vi "AbsMove.vi"(9 "Pos":dbl[](array[numeric]), 10 "error in":errorcluster) -> (2 "error out":errorcluster)   [LabVIEW 2022 SP3]
uses:
  Newport.XPS.CommandInterface
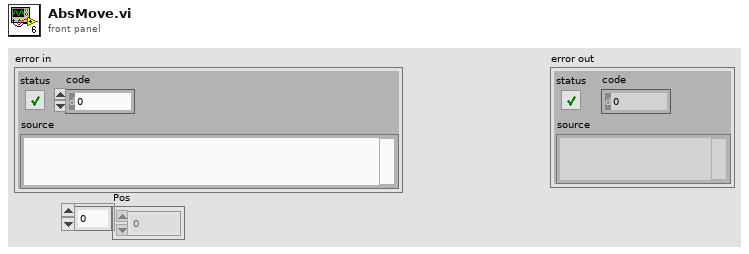
[diagram p1: front panel]
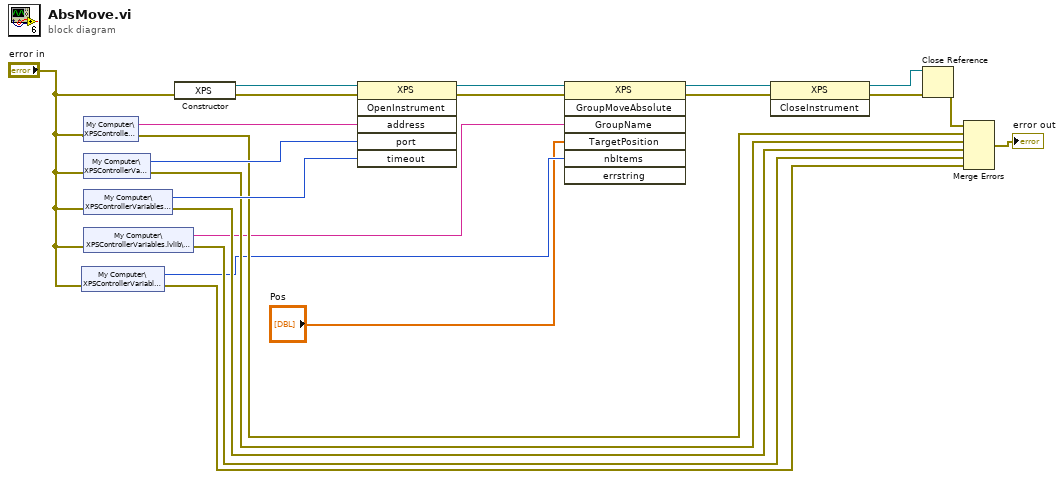
[diagram p0: block diagram]
diagram:
  n1 = shared-variable "My Computer\\XPSControllerVariables.lvlib\\nbitem"(error in="error in") -> (w4:i16, error out=w1:errorcluster)
  n2 = shared-variable "My Computer\\XPSControllerVariables.lvlib\\IP"(error in="error in") -> (w18:string, error out=w11:errorcluster)
  n3 = shared-variable "My Computer\\XPSControllerVariables.lvlib\\Port"(error in="error in") -> (w17:i16, error out=w10:errorcluster)
  n4 = shared-variable "My Computer\\XPSControllerVariables.lvlib\\Timeout"(error in="error in") -> (w16:i16, error out=w9:errorcluster)
  n5 = shared-variable "My Computer\\XPSControllerVariables.lvlib\\GroupName"(error in="error in") -> (w5:string, error out=w8:errorcluster)
  n6 = constructor class="XPS"(error in="error in") -> (reference out=w22:refnum<k24>, error out=w21:errorcluster)  [unwired: 2 in, 1 out]
  n7 = invoke class="XPS" method="OpenInstrument"(reference=w22, error in=w21, "address"=w18, "port"=w17, "timeout"=w16) -> (reference out=w20:refnum<k24>, error out=w19:errorcluster)  [unwired: 1 in, 4 out]
  n8 = invoke class="XPS" method="GroupMoveAbsolute"(reference=w20, error in=w19, "GroupName"=w5, "TargetPosition"="Pos", "nbItems"=w4) -> (reference out=w15:refnum<k24>, error out=w14:errorcluster)  [unwired: 2 in, 5 out]
  n9 = invoke class="XPS" method="CloseInstrument"(reference=w15, error in=w14) -> (reference out=w13:refnum<k24>, error out=w12:errorcluster)  [unwired: 1 in, 1 out]
  n10 = Close Reference(reference=w13, error in (no error)=w12) -> (error out=w7:errorcluster)
  n11 = Merge Errors(w7, w11, w10, w9, w8, w1) -> (→"error out":errorcluster)
